vi "Render.vi"(7 "Renderer":u32, 8 "error in (no error)":errorcluster, 10 "Camera":refnum<class "Camera.lvclass">, 11 "Planet in":refnum<class "Star.lvclass">) -> (0 "error out":errorcluster)   [LabVIEW 2021, in "Star.lvclass"]
uses:
  Star.lvclass
  Camera/Camera.lvclass
  Star.lvclass/Star.ctl
  Texture/Texture.lvclass
  C:/dev/LabVIEW/LabMelee/Source/Application Specific/Element/Element.lvclass
  C:/dev/LabVIEW/LabMelee/Source/Application Specific/Star/Star.lvclass
  Resource Manager/Resource Manager.lvclass
  Element/Element.lvclass
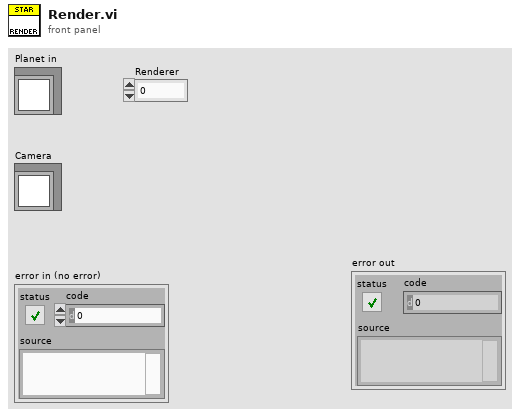
[diagram p1: front panel]
types:
  T1 = typedef "Camera.lvclass/Zoom Level.ctl" = enum16{"Far", "Medium", "Close"}
  T2 = typedef "SDL2 Utility.lvlib/Point (I32).ctl" = cluster{"x":i32, "y":i32}
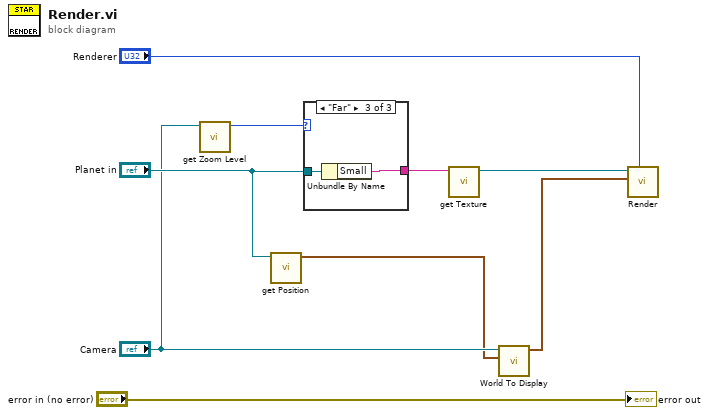
[diagram p0: block diagram]
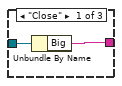
[diagram p2: hidden frame]
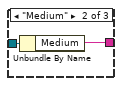
[diagram p3: hidden frame]
diagram:
  n1 = call "get Zoom Level.vi"("Camera in"="Camera") -> ("Zoom Level"=w7:T1)  [unwired: 10 in]
  n2 = call "get Position.vi"("Element in"="Planet in") -> ("Position"=w4:T2)  [unwired: 10 in]
  n3 = case shown="\"Far\"" w7 {
    tunnel: [w11 w13 w15] -> w8
    tunnel: "Planet in" -> [w10 w12 w14]
    frame "Close" {
      n4 = Unbundle By Name(w10) -> ("Big"=w11:string)
    }
    frame "Medium" {
      n5 = Unbundle By Name(w12) -> ("Medium"=w13:string)
    }
    frame "Far" {
      n6 = Unbundle By Name(w14) -> ("Small"=w15:string)
    }
  }
  n7 = call "get Texture.vi"("Texture Name"=w8) -> ("Texture"=w9:refnum<class "Texture.lvclass">)  [unwired: 10 in]
  n8 = call "World To Display.vi"("World Position"=w4, "Camera in"="Camera") -> ("Display Position"=w3:T2)  [unwired: 9 in]
  n9 = call-dynamic "Render.vi"("Renderer"="Renderer", "Destination"=w3, "Texture in"=w9) -> ()  [unwired: 9 in]
  "error out" <- "error in (no error)"
